vi "设计性实验-伏安特性曲线.vi"() -> ()   [LabVIEW 2021]
panel:
  out "Numeric 2":dbl
  out "Numeric":dbl
  out "XY Graph":cluster{"Y":dbl[], "Y":dbl[]}[](graph)
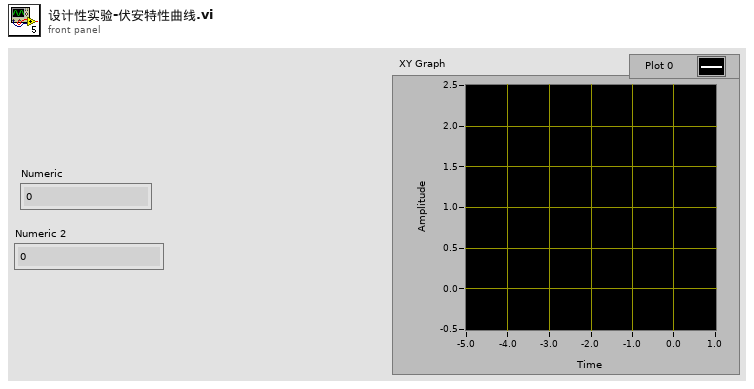
[diagram p1: front panel]
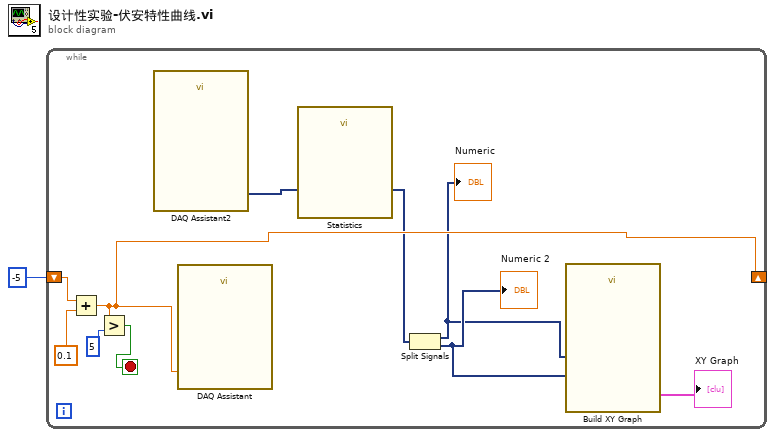
[diagram p0: block diagram]
diagram:
  n1 = while {
    shift-right: [w6] -> _
    shift-left: -5 -> [w10]
    stop <- w7 stop-if-true
    n2 = Add(x=w10, y=0.1) -> (x+y=w6:dbl)
    n3 = Greater?(x=w6, y=5) -> (0:w7:bool)
    n4 = call "DAQ Assistant2"() -> ("data"=w4:dynamicdata)  [unwired: 17 in, 2 out]
    n5 = call "DAQ Assistant"("data"=w6) -> ()  [unwired: 17 in, 2 out]
    n6 = call "Statistics"() -> ()  [unwired: 26 in, 2 out]
    n7 = Split Signals(w4) -> (w2:dynamicdata, w3:dynamicdata)  [unwired: 2 in]
    "Numeric" <- w2
    "Numeric 2" <- w3
    n8 = call "Build XY Graph"("Y Input"=w3, "X Input"=w2) -> ("XY Graph"=→"XY Graph":cluster{"X":dbl[], "Y":dbl[]}[])  [unwired: 8 in, 1 out]
  }
